vi "View Song Library Request.vi"(8 "error in (no error)":errorcluster, 11 "MusicManagerActor in":refnum<class "MusicManagerActor.lvclass">) -> (0 "error out":errorcluster, 3 "MusicManagerActor out":refnum<class "MusicManagerActor.lvclass">)   [LabVIEW 2015, in "MusicManagerActor.lvlib" / "MusicManagerActor.lvclass"]
uses:
  MusicManagerActor.lvclass
  MusicManagerActor.lvclass/MusicManagerActor.ctl
  SongBrowserActor/SongBrowserActor Messages/Display Song Library Msg/Display Song Library Msg.lvclass
  SongQueueActor/SongQueueActor Messages/Set Visibility Of Queue List Msg/Set Visibility Of Queue List Msg.lvclass
  file/MusicElement/MusicElementLibrary/MusicLibrary/MusicLibrary.lvclass
  file/MusicElement/MusicElementLibrary/SongLibrary/SongLibrary.lvclass
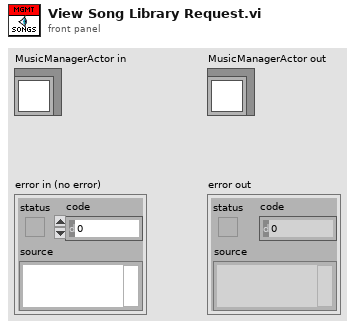
[diagram p1: front panel]
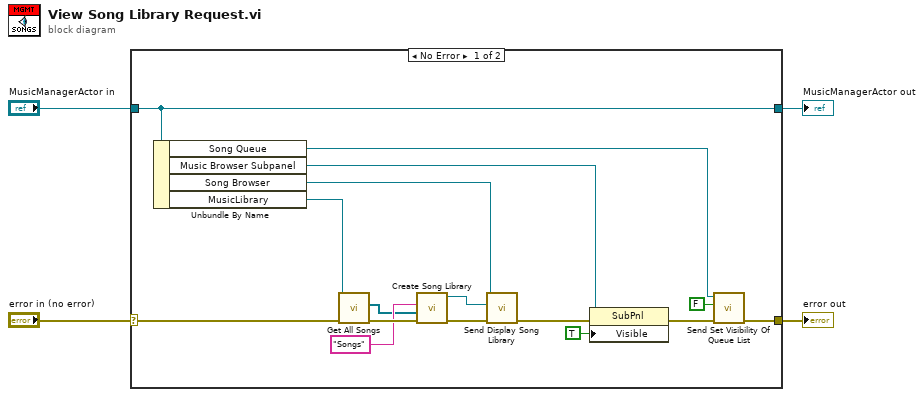
[diagram p0: block diagram]
diagram:
  n1 = case shown="No Error" "error in (no error)" {
    selector: "error in (no error)" -> [w11 w22]
    tunnel: [w13 w22] -> w3
    tunnel: [w20 w21] -> w1
    tunnel: "MusicManagerActor in" -> [w20 w21]
    frame No Error {
      n2 = Unbundle By Name(w20) -> ("Song Queue"=w12:refnum<class "Message Enqueuer.lvclass">, "Music Browser Subpanel"=w17:refnum<vi>, "Song Browser"=w19:refnum<class "Message Enqueuer.lvclass">, "MusicLibrary"=w10:refnum<class "MusicLibrary.lvclass">)
      n3 = call "Get All Songs.vi"("error in (no error)"=w11, "MusicLibrary in"=w10) -> ("error out"=w9:errorcluster, "Songs"=w7:refnum<class "Song.lvclass">[])  [unwired: 7 in, 1 out]
      n4 = call "Create Song Library.vi"("error in (no error)"=w9, "Songs"=w7, "Name"="Songs") -> ("error out"=w5:errorcluster, "SongLibrary out"=w6:refnum<class "SongLibrary.lvclass">)  [unwired: 7 in]
      n5 = call "Send Display Song Library.vi"("error in (no error)"=w5, "Song Library"=w6, "Message Enqueuer in"=w19) -> ("error out"=w18:errorcluster)  [unwired: 7 in, 1 out]
      n6 = property class="SubPnl"(reference=w17, error in=w18, "Visible"=TRUE) -> (error out=w14:errorcluster)  [unwired: 1 out]
      n7 = call "Send Set Visibility Of Queue List.vi"("error in (no error)"=w14, "Visible"=FALSE, "Message Enqueuer in"=w12) -> ("error out"=w13:errorcluster)  [unwired: 7 in, 1 out]
    }
    frame Error {
    }
  }
  "error out" <- w3
  "MusicManagerActor out" <- w1
